vi "Step 3.vi"(8 "error in (no error)":errorcluster, 11 "HeatUp Data in":string[][](array[string])) -> (0 "error out":errorcluster, 2 "Final Discharge Temperature":dbl format="%.2f", 3 "Max Temp Difference":dbl, 4 "Raw Data (Final Discharge and Compressor Shell)":string[][](array[string]), 5 "Raw Data (Temp Difference)":string[][](array[string]))   [LabVIEW 2019]
uses:
  <vilib>/Utility/error.llb/DialogType.ctl
panel:
  out "element":i32
  out "Min Temp Difference":dbl
  out "HeatUp Data in 2":string[][](array[string])
  # "Data with Stripped Header"
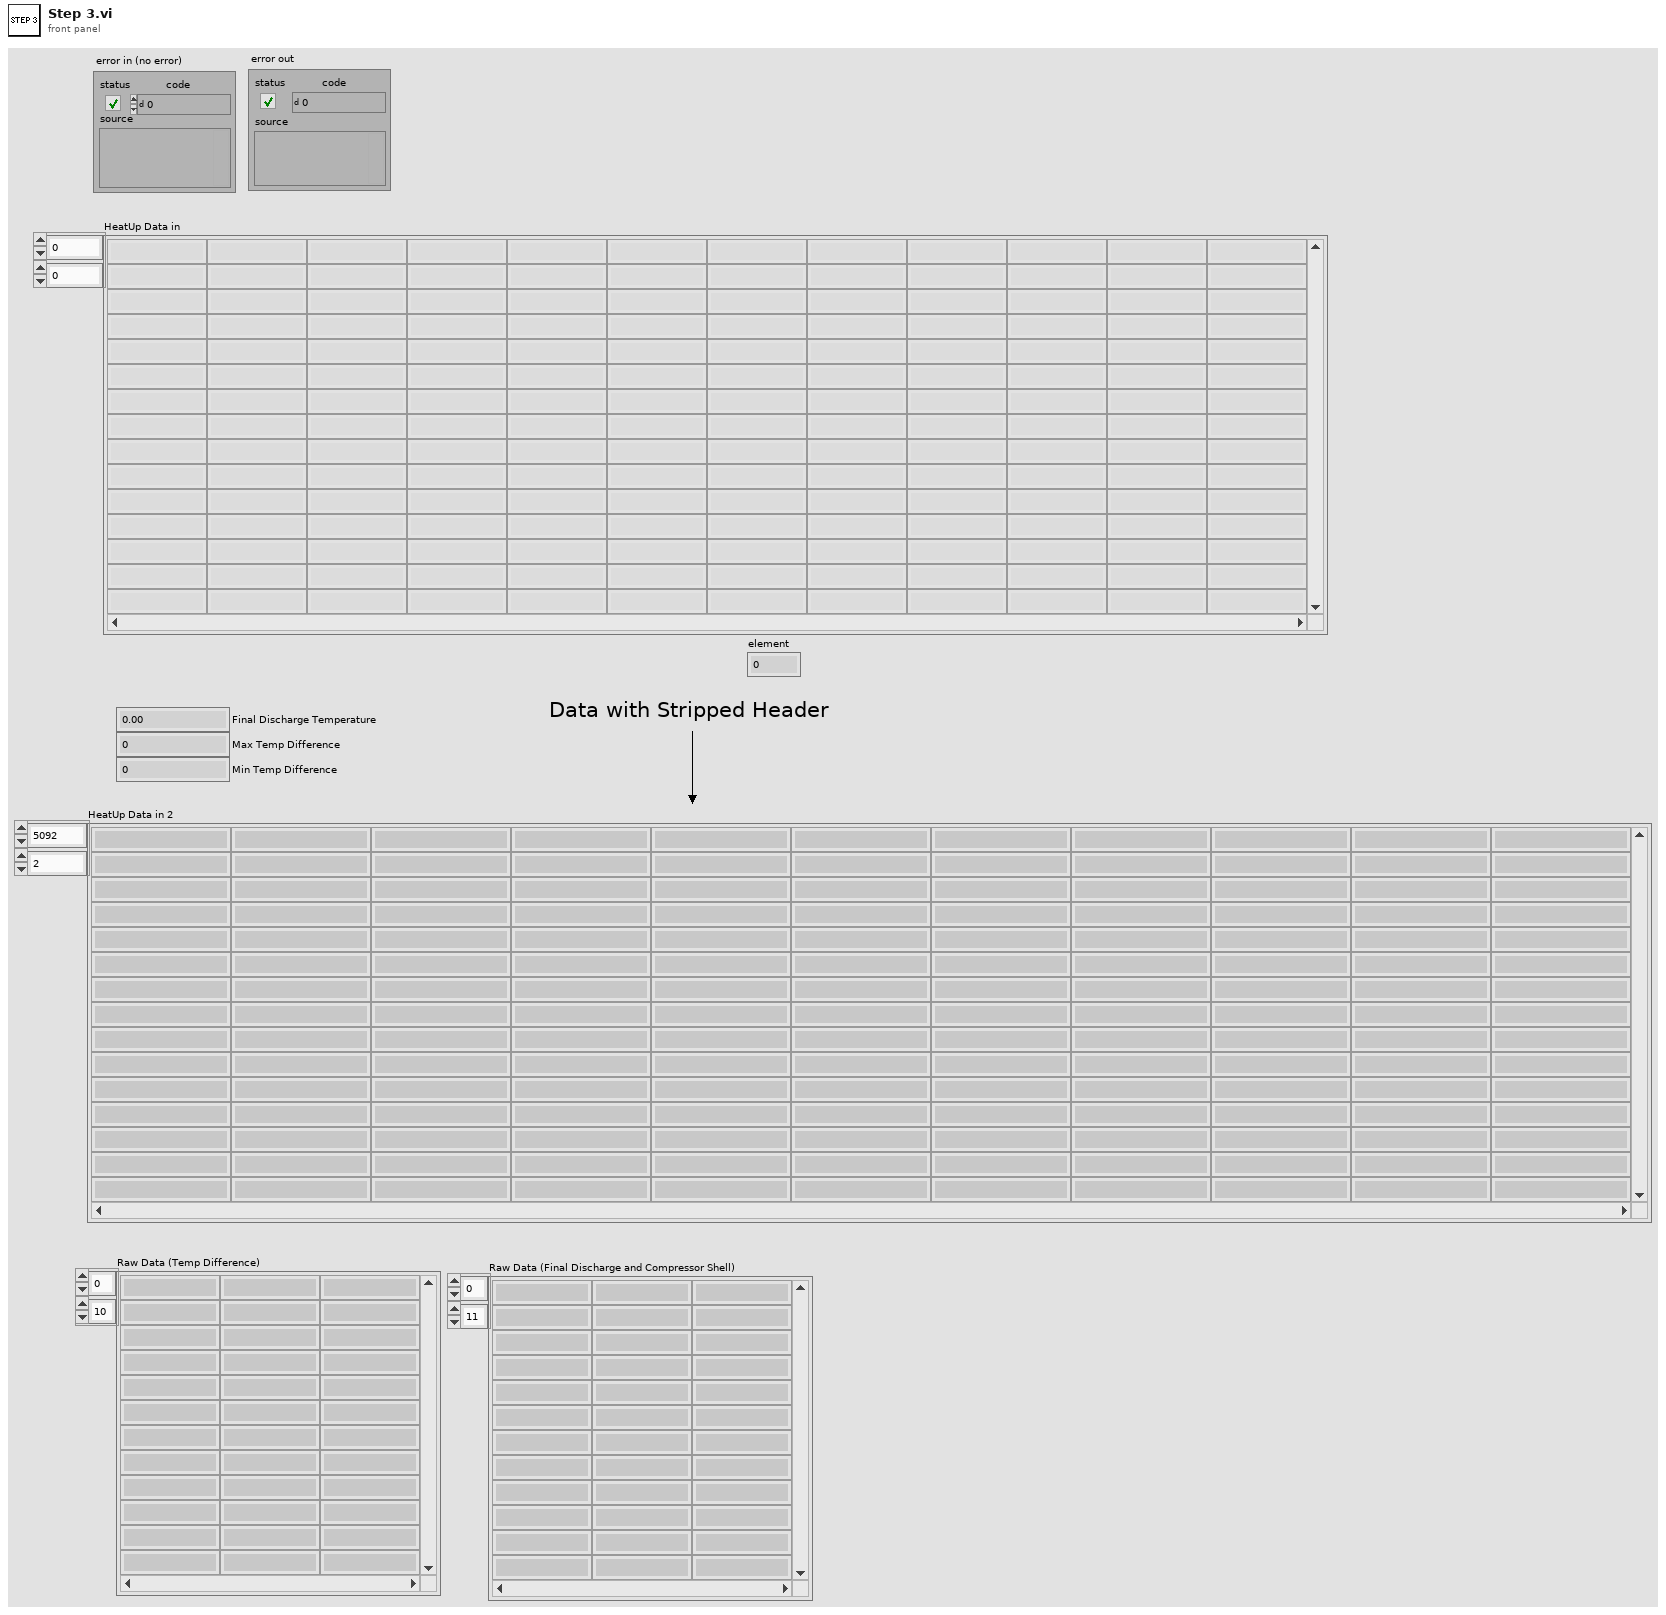
[diagram p1: front panel]
types:
  T1 = typedef "DialogType.ctl" = u16
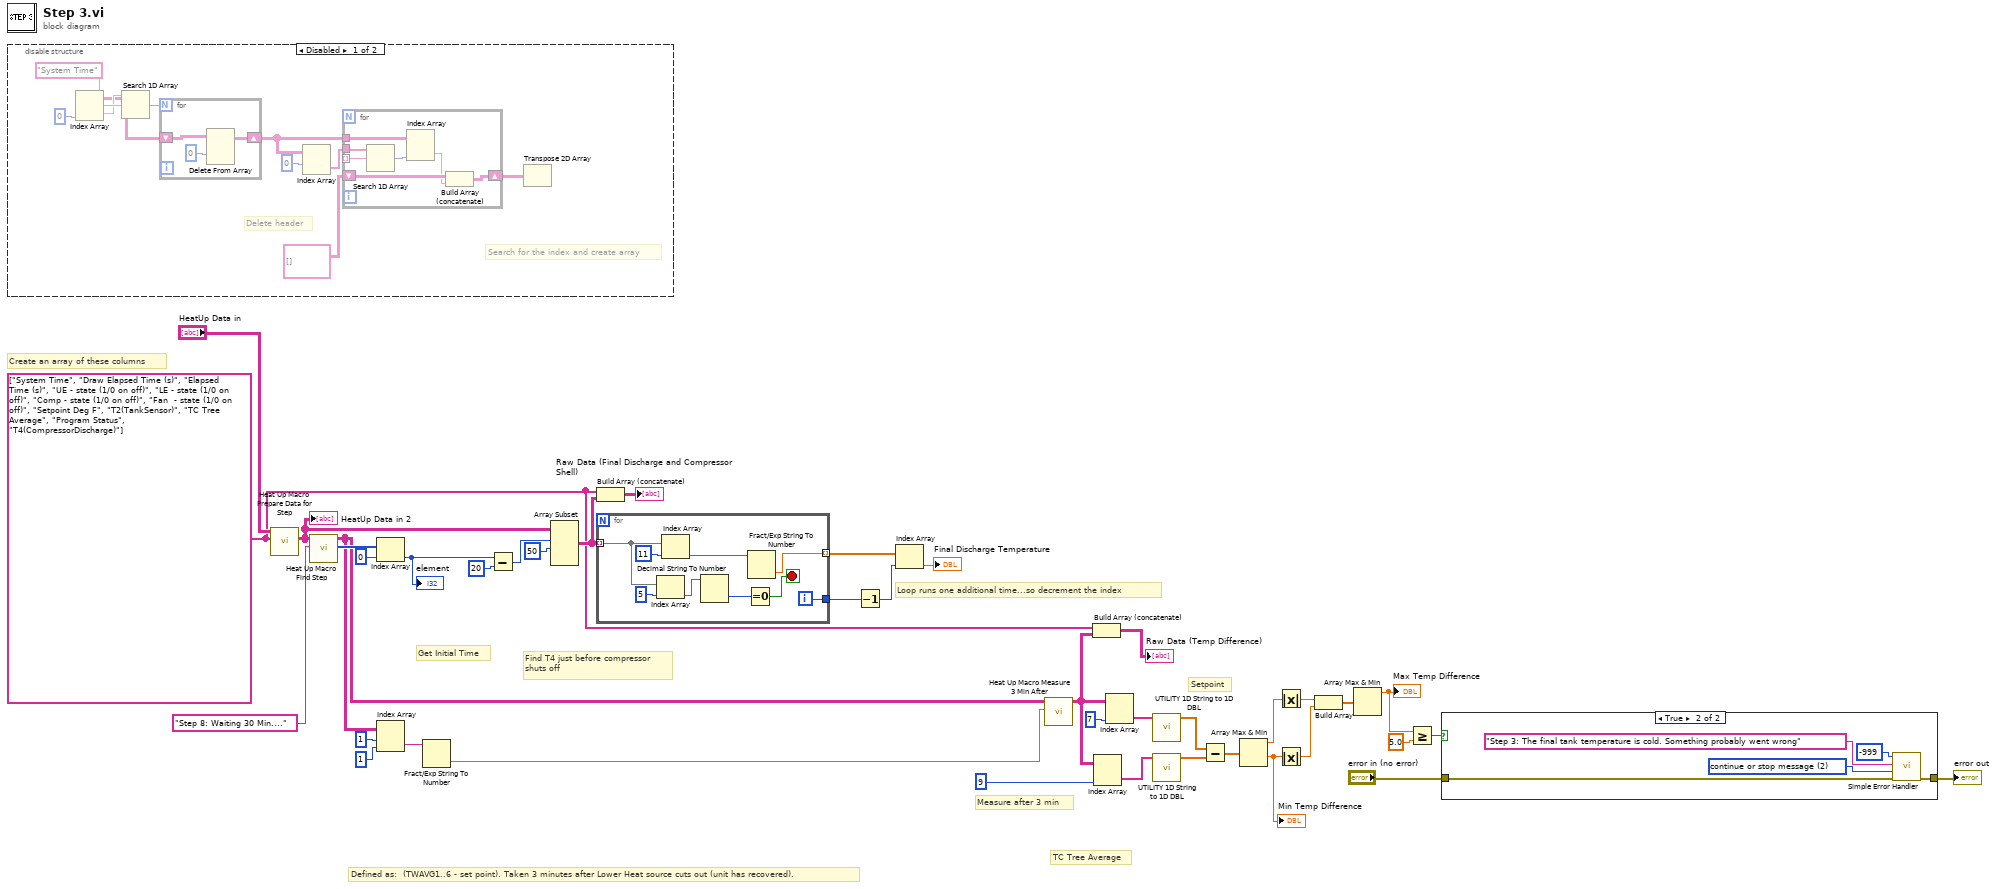
[diagram p0: block diagram]
diagram:
  w7 = string[] ["System Time", "Draw Elapsed Time (s)", "Elapsed Time (s)", "UE - state (1/0 on off)", "LE - state (1/0 on off)", "Comp - state (1/0 on off)", "Fan  - state (1/0 on off)", "Setpoint Deg F", "T2(TankSensor)", "TC Tree Average", "Program Status", "T4(CompressorDischarge)"]
  # "Loop runs one additional time...so decrement the index"
  # "Find T4 just before compressor\nshuts off"
  # "Measure after 3 min"
  # "TC Tree Average"
  # "Setpoint"
  # "Get Initial Time"
  # "Defined as:  (TWAVG1..6 - set point). Taken 3 minutes after Lower Heat source cuts out (unit has recovered)."
  # "Create an array of these columns"
  n1 = disable-structure shown="Disabled" {
    frame Disabled {
      # "Delete header"
      # "Search for the index and create array"
      n2 = Index Array(index (col)=0 ("disabled index (col)")) -> (array=w41:string[][], element=w48)  [unwired: 1 in]
      n3 = Search 1D Array(1D array=w48, element="System Time") -> (index of element=w50:i32)  [unwired: 1 in]
      n4 = for {
        N: w50 -> [_]
        shift-right: [w59] -> w43
        shift-left: w41 -> [w60]
        n5 = Delete From Array(array=w60, index (row)=0) -> (array with subset deleted=w59:string[][])  [unwired: 2 in, 1 out]
      }
      n6 = Index Array(array=w43, index (row)=0) -> (element=w45:string[])  [unwired: 1 in]
      n7 = for {
        tunnel: w45 -> [w57]
        tunnel: _ -> [w56] mode=indexing
        shift-right: [w54] -> w42
        shift-left: string[][] [] -> [w55]
        tunnel: w43 -> [w53]
        n8 = Search 1D Array(1D array=w57, element=w56) -> (index of element=w52:i32)  [unwired: 1 in]
        n9 = Index Array(array=w53, index (col)=w52) -> (element=w51:string[])  [unwired: 1 in]
        n10 = Build Array (concatenate)(w55, w51) -> (w54:string[][])
      }
      n11 = Transpose 2D Array(2D array=w42) -> ()  [unwired: 1 out]
    }
    frame Enabled {
    }
  }
  n12 = call "Heat Up Macro Prepare Data for Step.vi"("Columns Too Search For"=w7, "HeatUp Raw Data Input"="HeatUp Data in") -> ("Heat Up Data with Only Selected Columns"=w5:string[][])  [unwired: 8 in, 1 out]
  "HeatUp Data in 2" <- w5
  n13 = call "Heat Up Macro Find Step.vi"("Search For Step Name"="Step 8: Waiting 30 Min...." ("y"), "Heat Up Data with Only Selected Columns"=w5) -> ("Index"=w4:i32[], "Filtered Array"=w3:string[][])  [unwired: 7 in, 1 out]
  n14 = Index Array(array=w4, index=0) -> (element=w19:i32)
  "element" <- w19
  n15 = Index Array(array=w3, index (row)=1 ("index"), index (col)=1 ("disabled index (col)")) -> (element=w28:string)
  n16 = Fract/Exp String To Number(string=w28) -> (number=w2:dbl)  [unwired: 3 in, 1 out]
  n17 = Subtract(x=w19, y=20) -> (x-y=w17:i32)
  n18 = Array Subset(array=w5, index (row)=w17, length (row)=50 ("length")) -> (w11:string[][])  [unwired: 2 in]
  n19 = Build Array (concatenate)(w7, w11) -> (→"Raw Data (Final Discharge and Compressor Shell)":string[][])
  n20 = for {
    tunnel: w11 -> [w61] mode=indexing
    tunnel: [w62] -> w15 mode=indexing
    tunnel: [w64] -> w13
    i -> [w64]
    stop <- w66 stop-if-true
    n21 = Index Array(array=w61, index=5) -> (element=w68:string)
    n22 = Index Array(array=w61, index=11) -> (element=w63:string)
    n23 = Decimal String To Number(string=w68) -> (number=w67:i32)  [unwired: 2 in, 1 out]
    n24 = Equal To 0?(x=w67) -> (x = 0?=w66:bool)
    n25 = Fract/Exp String To Number(string=w63) -> (number=w62:dbl)  [unwired: 3 in, 1 out]
  }
  n26 = Decrement(x=w13) -> (x-1=w12:i32)
  n27 = Index Array(array=w15, index=w12) -> (element=→"Final Discharge Temperature":dbl)
  n28 = call "Heat Up Macro Measure 3 Min After.vi"("Start Time"=w2, "Array in"=w3) -> ("Array out"=w1:string[][])  [unwired: 9 in]
  n29 = Build Array (concatenate)(w7, w1) -> (→"Raw Data (Temp Difference)":string[][])
  n30 = Index Array(array=w1, index (col)=9 ("disabled index (col)")) -> (element=w37:string[])  [unwired: 1 in]
  n31 = Index Array(array=w1, index (col)=7 ("disabled index (col)")) -> (element=w38:string[])  [unwired: 1 in]
  n32 = call "UTILITY 1D String to 1D DBL.vi"("Save Data"=w38) -> ("DBL"=w36:dbl[])  [unwired: 10 in]
  n33 = call "UTILITY 1D String to 1D DBL.vi"("Save Data"=w37) -> ("DBL"=w35:dbl[])  [unwired: 10 in]
  n34 = Subtract(x=w36, y=w35) -> (x-y=w34:dbl[])
  n35 = Array Max & Min(array=w34) -> (max value=w33:dbl, min value=w32:dbl)  [unwired: 2 out]
  "Min Temp Difference" <- w32
  n36 = Absolute Value(x=w33) -> (abs(x)=w30:dbl)
  n37 = Absolute Value(x=w32) -> (abs(x)=w31:dbl)
  n38 = Build Array(w30, w31) -> (w29:dbl[])
  n39 = Array Max & Min(array=w29) -> (max value=w21:dbl)  [unwired: 3 out]
  "Max Temp Difference" <- w21
  n40 = Greater Or Equal?(x=w21, y=5.0) -> (x >= y?=w25:bool)
  n41 = case shown="True" w25 {
    tunnel: "error in (no error)" -> [w70 w75]
    tunnel: [w70 w74] -> w22
    frame False {
    }
    frame True {
      w73 = T1 2 items=["no dialog", "OK message", "continue or stop message", "OK message + warnings", "continue/stop + warnings"] ("type of dialog (OK msg:1)")
      n42 = call <vilib>:"Simple Error Handler.vi"("error code (no error:0)"=-999, "error source (\" \")"="Step 3: The final tank temperature is cold. Something probably went wrong" ("error source (\" \")"), "type of dialog (OK msg:1)"=w73, "error in (no error)"=w75) -> ("error out"=w74:errorcluster)  [unwired: 1 in, 4 out]
    }
  }
  "error out" <- w22
